vi "Fgen Module.vi"() -> ()   [LabVIEW 2021]
uses:
  <instrlib>/niScope/Acquire/niScope Multi Read Cluster.vi
panel:
  in  "Channel(s)":string="0" caption="Scope Channel(s)"
  in  "resource name":refnum<k15>="Dev1" caption="Scope"
  out "Waveform Graph":T1(graph)
  in  "duration":dbl
  out "Actual Duration":dbl
  in  "I2C Generator Fgen":refnum<k15>
  in  "amplitude":dbl=6.0
  in  "frequency":dbl=6.0
  in  "waveform":T2(ring)=enum."Noise"
  in  "I2C Generator Fgen Channel":string
  out "error out":errorcluster
  in  "error in":errorcluster
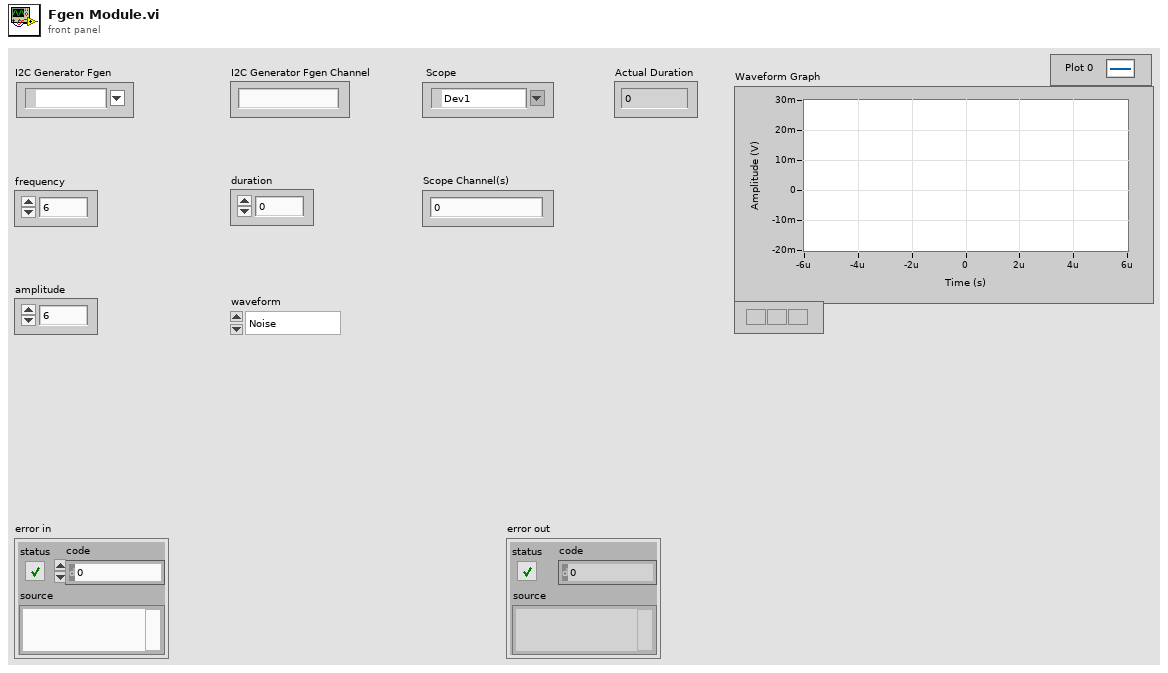
[diagram p1: front panel]
types:
  T1 = cluster{"relativeInitialX":dbl, "xIncrement":dbl, "wfm":dbl[]}[]
  T2 = enum32{"Sine", "Square", "Triangle", "Ramp Up", "Ramp Down", "DC", "Noise", "User"}
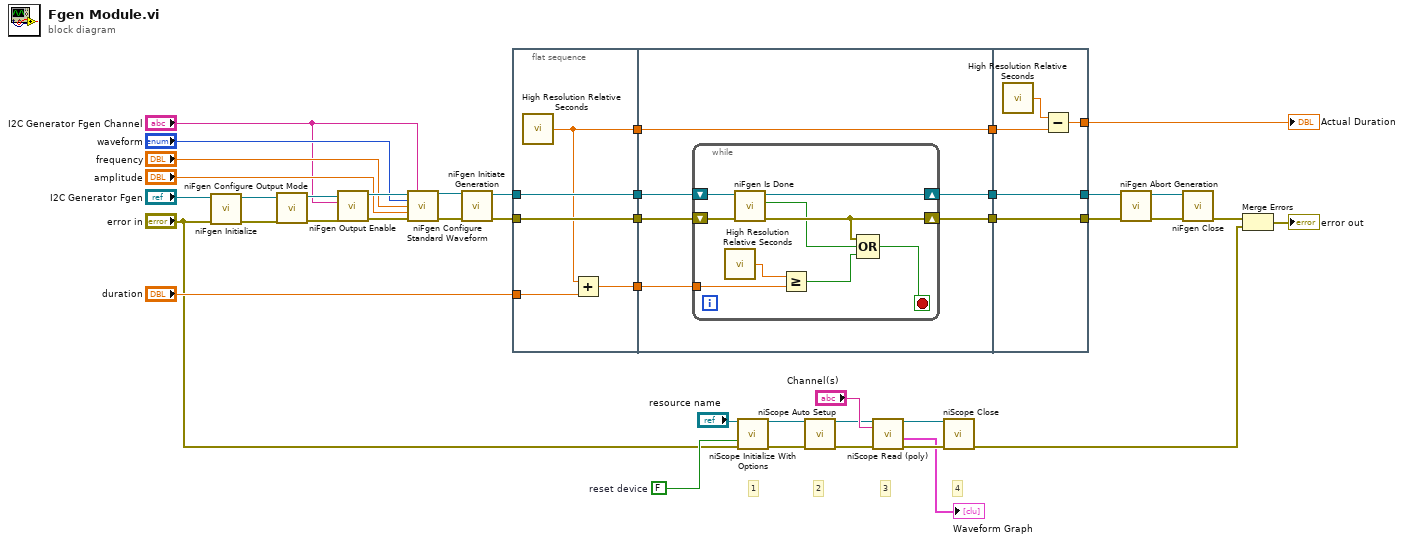
[diagram p0: block diagram]
diagram:
  w7 = FALSE  # reset device
  # "4"
  # "3"
  # "2"
  # "1"
  n1 = call <instrlib>:"niFgen Initialize.vi"("error in (no error)"="error in", "Resource Name"="I2C Generator Fgen") -> ("error out"=w39:errorcluster, "Instrument Handle Out"=w42:refnum<k15>)  [unwired: 8 in]
  n2 = call <instrlib>:"niFgen Configure Output Mode.vi"("error in (no error)"=w39, "Instrument Handle"=w42) -> ("error out"=w28:errorcluster, "Instrument Handle Out"=w38:refnum<k15>)  [unwired: 7 in]
  n3 = call <instrlib>:"niFgen Output Enable.vi"("error in (no error)"=w28, "Channel Name"="I2C Generator Fgen Channel", "Instrument Handle"=w38) -> ("error out"=w40:errorcluster, "Instrument Handle Out"=w37:refnum<k15>)  [unwired: 7 in]
  n4 = call <instrlib>:"niFgen Configure Standard Waveform.vi"("Instrument Handle"=w37, "Channel Name"="I2C Generator Fgen Channel", "Waveform"="waveform", "Frequency"="frequency", "Amplitude"="amplitude", "error in (no error)"=w40) -> ("Instrument Handle Out"=w36:refnum<k15>, "error out"=w41:errorcluster)  [unwired: 8 in]
  n5 = call <instrlib>:"niFgen Initiate Generation.vi"("error in (no error)"=w41, "Instrument Handle"=w36) -> ("error out"=w33:errorcluster, "Instrument Handle Out"=w35:refnum<k15>)  [unwired: 8 in]
  n6 = flat-sequence {
    tunnel: w33 -> [w46]
    tunnel: w35 -> [w47]
    tunnel: [w47] -> w22
    tunnel: [w46] -> w21
    tunnel: [w45] -> w17
    tunnel: "duration" -> [w44]
    tunnel: [w43] -> w14
    tunnel: w22 -> [w53]
    tunnel: w21 -> [w51]
    tunnel: [w52] -> w20
    tunnel: [w50] -> w19
    tunnel: [w49] -> w18
    tunnel: w17 -> [w49]
    tunnel: w14 -> [w48]
    tunnel: [w66] -> w32
    tunnel: [w67] -> w34
    tunnel: w20 -> [w67]
    tunnel: w19 -> [w66]
    tunnel: w18 -> [w64]
    tunnel: [w63] -> w16
    frame #0 {
      n7 = call <vilib>:"High Resolution Relative Seconds.vi"() -> ("relative seconds"=w45:dbl)
      n8 = Add(x=w45, y=w44) -> (x+y=w43:dbl)
    }
    frame #1 {
      n9 = while {
        shift-right: [w61] -> w52
        shift-left: w53 -> [w62]
        shift-right: [w59] -> w50
        shift-left: w51 -> [w60]
        tunnel: w48 -> [w56]
        stop <- w58 stop-if-true
        n10 = call <vilib>:"High Resolution Relative Seconds.vi"() -> ("relative seconds"=w57:dbl)
        n11 = call <instrlib>:"niFgen Is Done.vi"("error in (no error)"=w60, "Instrument Handle"=w62) -> ("error out"=w59:errorcluster, "Done"=w54:bool, "Instrument Handle Out"=w61:refnum<k15>)  [unwired: 7 in]
        n12 = Greater Or Equal?(x=w57, y=w56) -> (x >= y?=w55:bool)
        n13 = Compound Arithmetic op=OR(w59, w54, w55) -> (w58:bool)
      }
    }
    frame #2 {
      n14 = call <vilib>:"High Resolution Relative Seconds.vi"() -> ("relative seconds"=w65:dbl)
      n15 = Subtract(x=w65, y=w64) -> (x-y=w63:dbl)
    }
  }
  n16 = call <instrlib>:"niScope Initialize With Options.vi"("resource name"="resource name", "reset device"=w7, "error in"="error in") -> ("instrument handle"=w4:refnum<k15>, "error out"=w5:errorcluster)  [unwired: 11 in]
  n17 = call <instrlib>:"niScope Auto Setup.vi"("instrument handle"=w4, "error in"=w5) -> ("instrument handle out"=w8:refnum<k15>, "error out"=w9:errorcluster)  [unwired: 12 in]
  n18 = call-poly <instrlib>:"niScope Read (poly).vi"("error in"=w9, "channels"="Channel(s)", "instrument handle"=w8) -> ("error out"=w12:errorcluster, "waveform"=→"Waveform Graph":T1, "instrument handle out"=w13:refnum<k15>)  [unwired: 5 in, 1 out]
  n19 = call <instrlib>:"niScope Close.vi"("instrument handle"=w13, "error in"=w12) -> ("error out"=w1:errorcluster)  [unwired: 13 in]
  n20 = call <instrlib>:"niFgen Abort Generation.vi"("error in (no error)"=w32, "Instrument Handle"=w34) -> ("error out"=w30:errorcluster, "Instrument Handle Out"=w31:refnum<k15>)  [unwired: 8 in]
  n21 = call <instrlib>:"niFgen Close.vi"("error in (no error)"=w30, "Instrument Handle"=w31) -> ("error out"=w29:errorcluster)  [unwired: 9 in]
  n22 = Merge Errors(w29, w1) -> (→"error out":errorcluster)
  "Actual Duration" <- w16
